vi "DCA Compute Pi-Attenuation.vi"(1 "Measurement Values":T1) -> (0 "Pi-Attenuation":dbl)   [LabVIEW 2011]
uses:
  TypeDefs/DCA Measurement Values.ctl
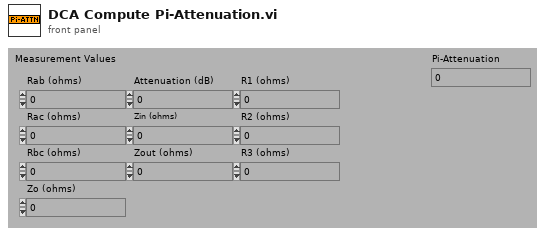
[diagram p1: front panel]
types:
  T1 = typedef "DCA Measurement Values.ctl" = cluster{"Rab (ohms)":dbl, "Rac (ohms)":dbl, "Rbc (ohms)":dbl, "Zo (ohms)":dbl, "Attenuation (dB)":dbl, "Zin (ohms)":dbl, "Zout (ohms)":dbl, "R1 (ohms)":dbl, "R2 (ohms)":dbl, "R3 (ohms)":dbl}
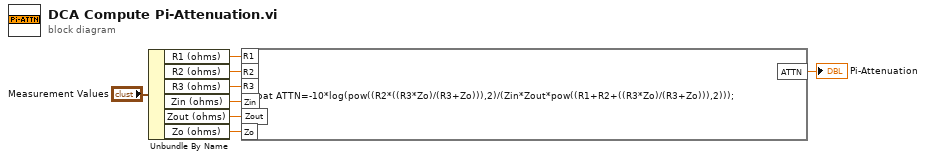
[diagram p0: block diagram]
diagram:
  n1 = Unbundle By Name("Measurement Values") -> ("R1 (ohms)"=w7:dbl, "R2 (ohms)"=w6:dbl, "R3 (ohms)"=w5:dbl, "Zin (ohms)"=w3:dbl, "Zout (ohms)"=w2:dbl, "Zo (ohms)"=w1:dbl)
  n2 = formula code="float ATTN=-10*log(pow((R2*((R3*Zo)/(R3+Zo))),2)/(Zin*Zout*pow((R1+R2+((R3*Zo)/(R3+Zo))),2)));"("R1"=w7, "R2"=w6, "R3"=w5, "Zin"=w3, "Zout"=w2, "Zo"=w1) -> ("ATTN"=→"Pi-Attenuation":dbl)
